vi "Router Example.vi"() -> ()   [LabVIEW 2016, in "PXImc Custom Device Engine.lvlib" / "PXImc Router.lvlib"]
uses:
  Shared/PXImc Router/Controls/Router - Configuration.ctl
  Shared/PXImc Router/Controls/Node Properties.ctl
  Shared/PXImc Router/Controls/Table Index-Size.ctl
  <vilib>/Utility/error.llb/DialogType.ctl
  Shared/PXImc Router/VIs/Router/Router - Globals.vi
  PXImc Router.lvlib
  Shared/PXImc Router/PXImc Router.lvlib
panel:
  out "Array":dbl[](array[numeric])=[1.0, 2.0, 3.0, 4.0, 5.0, 11.0, 12.0, 13.0, 14.0, 15.0]
  out "Waveform Chart":T1(graph)={"[0]"=1.0, "[1]"=2.0, "[2]"=3.0, "[3]"=4.0, "[4]"=5.0, "[5]"=11.0, "[6]"=12.0, "[7]"=13.0, "[8]"=14.0}
  in  "stop":bool
  in  "Router - Configuration Properties":T2={"Node Properties"=[{"Resource Name"="PXI1Slot2", "Slave IP Address"="", "Node ID"=1, "Node # Channels"=5, "Reading Segments"={"Index"=0, "Size"=5}, "Writing Segments"=[{"Index"=5, "Size"=5}]}, {"Resource Name"="PXI1Slot2", "Slave IP Address"="", "Node ID"=2, "Node # Channels"=5, "Reading Segments"={"Index"=5, "Size"=5}, "Writing Segments"=[{"Index"=0, "Size"=5}]}], "Connection Timeout (s)"=60.0, "Readers Buffer Size"=250000}
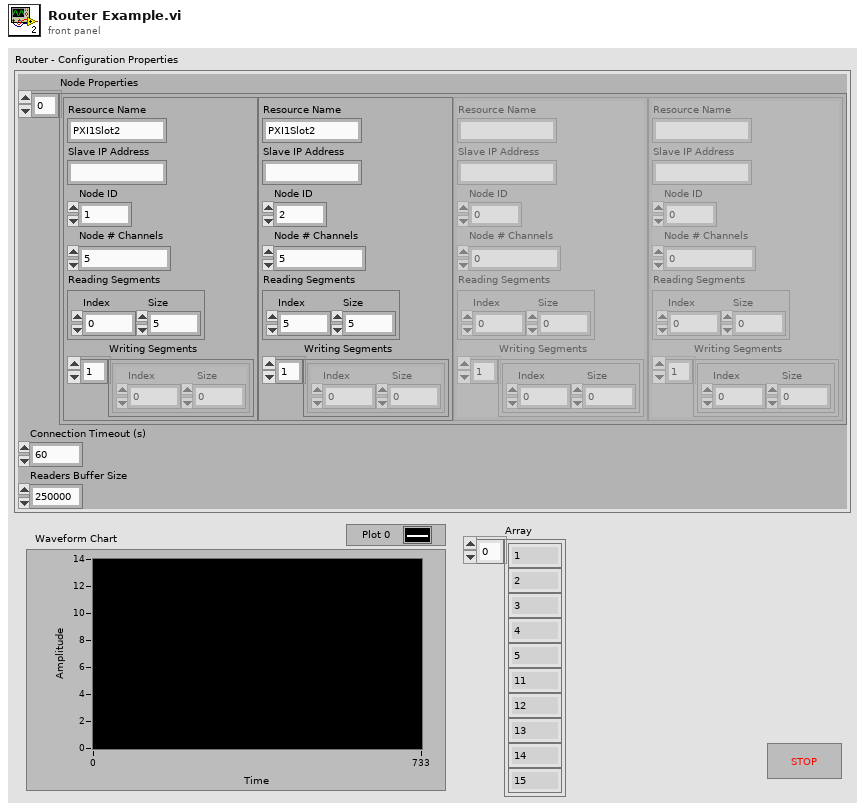
[diagram p1: front panel]
types:
  T1 = cluster{"[0]":dbl, "[1]":dbl, "[2]":dbl, "[3]":dbl, "[4]":dbl, "[5]":dbl, "[6]":dbl, "[7]":dbl, "[8]":dbl}
  T2 = typedef "PXImc Router.lvlib/Router - Configuration.ctl" = cluster{"Node Properties":T3[], "Connection Timeout (s)":dbl, "Readers Buffer Size":u32}
  T3 = typedef "PXImc Router.lvlib/Node Properties.ctl" = cluster{"Resource Name":string, "Slave IP Address":string, "Node ID":u16, "Node # Channels":u32, "Reading Segments":T4, "Writing Segments":T4[]}
  T4 = typedef "PXImc Router.lvlib/Table Index-Size.ctl" = cluster{"Index":u32, "Size":u32}
  T5 = typedef "DialogType.ctl" = u16
  T6 = typedef "PXImc Router.lvlib/Router Data.ctl" = cluster{"Master Table Ref":refnum<data-value>, "Reader Data":T7, "Writer Data":T8}
  T7 = typedef "PXImc Router.lvlib/Reader Data.ctl" = cluster{"Reader - Session Refs":refnum<k21>[], "Reading Segments":T4[]}
  T8 = typedef "PXImc Router.lvlib/Writer Data.ctl" = cluster{"Writer - Session Refs":refnum<k21>[], "Writing Segments":T4[][]}
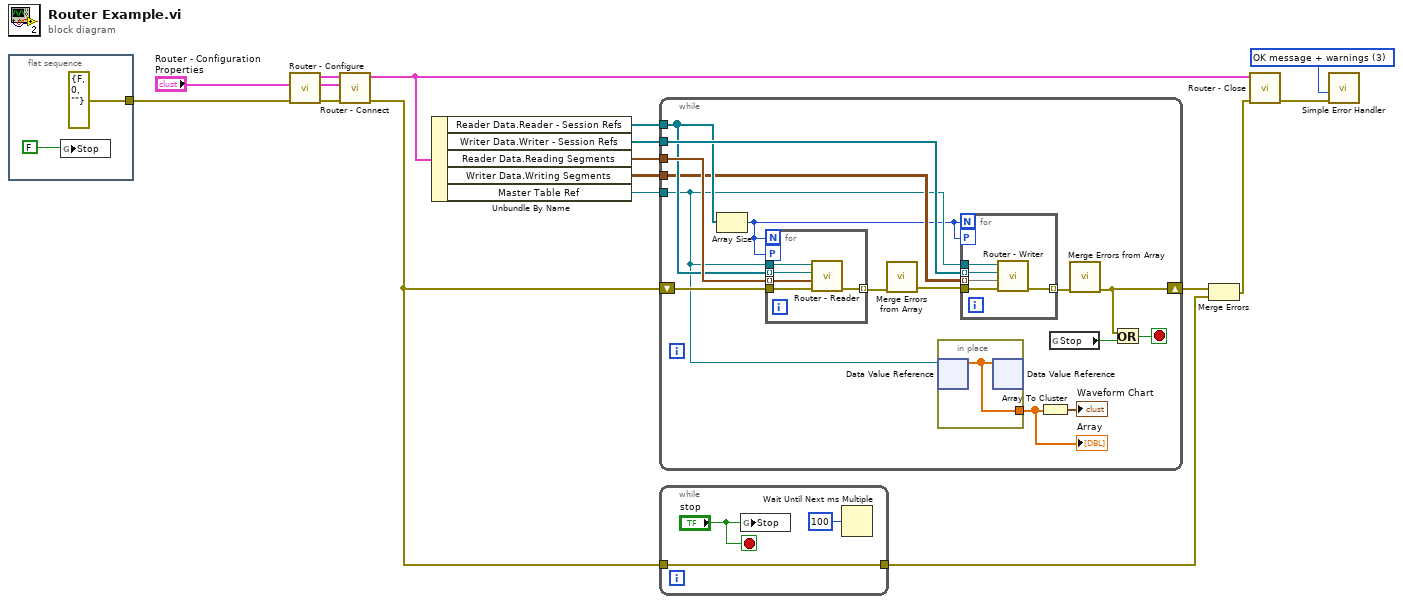
[diagram p0: block diagram]
diagram:
  w16 = T5 3 items=["no dialog", "OK message", "continue or stop message", "OK message + warnings", "continue/stop + warnings"] ("type of dialog (OK msg:1)")
  n1 = flat-sequence {
    tunnel: [errorcluster {"status"=FALSE, "code"=0, "source"=""} ("error constant")] -> w15
    frame #0 {
      n2 = global write "Router - Globals.vi" "Stop"(FALSE ("Stopped")) -> ()
    }
  }
  n3 = call "Router - Configure.vi"("error in (no error)"=w15, "Configuration Properties In"="Router - Configuration Properties") -> ("error out"=w4:errorcluster, "Configuration Properties Out"=w5:T2, "Router Data Out"=w6:T6)  [unwired: 7 in]
  n4 = call "Router - Connect.vi"("error in (no error)"=w4, "Configuration Properties"=w5, "Router Data In"=w6) -> ("error out"=w3:errorcluster, "Router Data Out"=w2:T6)  [unwired: 6 in, 1 out]
  n5 = Unbundle By Name(w2) -> ("Reader Data.Reader - Session Refs"=w9:refnum<k21>[], "Writer Data.Writer - Session Refs"=w8:refnum<k21>[], "Reader Data.Reading Segments"=w11:T4[], "Writer Data.Writing Segments"=w7:T4[][], "Master Table Ref"=w10:refnum<data-value>)
  n6 = while {
    tunnel: w10 -> [w23]
    tunnel: w9 -> [w25]
    tunnel: w8 -> [w26]
    tunnel: w11 -> [w34]
    shift-right: [w27] -> w12
    shift-left: w3 -> [w33]
    tunnel: w7 -> [w24]
    stop <- w32 stop-if-true
    n7 = Array Size(array=w25) -> (size(s)=w20:i32)
    n8 = for {
      N: w20 -> [_]
      workers-P: w20 -> [_]
      tunnel: w34 -> [w35] mode=indexing
      tunnel: w23 -> [w39]
      tunnel: w25 -> [w38] mode=indexing
      tunnel: w33 -> [w37]
      tunnel: [w36] -> w30 mode=indexing
      n9 = call "Router - Reader.vi"("error in (no error)"=w37, "Reading Segments"=w35, "PXImc Reading Session In"=w38, "Master Table Ref In"=w39) -> ("error out"=w36:errorcluster)  [unwired: 7 in]
    }
    n10 = call "Merge Errors from Array.vi"("Error Array In"=w30) -> ("error out"=w28:errorcluster)  [unwired: 10 in]
    n11 = in-place {
      in-place-border: [w45] -> w22
      n12 = in-place-dvr #1(w23) -> (w45:dbl[])  [unwired: 1 out]
      n13 = in-place-dvr #1(w45) -> ()  [unwired: 2 out]
    }
    "Array" <- w22
    n14 = for {
      N: w20 -> [_]
      tunnel: w23 -> [w44]
      tunnel: w26 -> [w41] mode=indexing
      tunnel: w28 -> [w43]
      tunnel: [w42] -> w29 mode=indexing
      tunnel: w24 -> [w40] mode=indexing
      workers-P: w20 -> [_]
      n15 = call "Router - Writer.vi"("error in (no error)"=w43, "Reading Segments Array"=w40, "PXImc Writing Session In"=w41, "Master Table Ref In"=w44) -> ("error out"=w42:errorcluster)  [unwired: 7 in]
    }
    n16 = Array To Cluster(array=w22) -> (cluster=→"Waveform Chart":T1)
    n17 = global read "Router - Globals.vi" "Stop"() -> (w31:bool)
    n18 = call "Merge Errors from Array.vi"("Error Array In"=w29) -> ("error out"=w27:errorcluster)  [unwired: 10 in]
    n19 = Or(x=w27, y=w31) -> (x .or. y?=w32:bool)
  }
  n20 = while {
    tunnel: w3 -> [w46]
    tunnel: [w46] -> w14
    stop <- "stop" stop-if-true
    n21 = global write "Router - Globals.vi" "Stop"("stop") -> ()
    n22 = Wait Until Next ms Multiple(millisecond multiple=u32 100) -> ()  [unwired: 1 out]
  }
  n23 = Merge Errors(w12, w14) -> (w13:errorcluster)
  n24 = call "Router - Close.vi"("error in (no error)"=w13, "Router Data"=w2) -> ("error out"=w17:errorcluster)  [unwired: 9 in]
  n25 = call <vilib>:"Simple Error Handler.vi"("type of dialog (OK msg:1)"=w16, "error in (no error)"=w17) -> ()  [unwired: 3 in, 5 out]
